vi "Example.Async.vi"() -> ()   [LabVIEW 2015, in "Inline Async Example Engine.lvlib"]
uses:
  Inline Async Example Engine.lvlib
  Inline Async APIs/VS Inline Async API/Process/Process.lvclass
  Inline Async APIs/Data Access Engine/Data Access Engine.lvclass
  Inline Async APIs/Data Access Engine/Data/Read/Read.lvclass/Read.ctl
  Inline Async APIs/Data Access Engine/Data/Write/Write.lvclass/Write.ctl
  Inline Async APIs/VS Inline Async API/Process/Process.lvclass/Process.ctl
  Inline Async APIs/Data Access Engine/Methods/Read.Data.vi
  Inline Async APIs/Data Access Engine/Methods/Write.Data.vi
  Inline Async APIs/Data Access Engine/Data/Read/Read.ProcessData.vi
  Inline Async APIs/Data Access Engine/Data/Write/Write.ProcessData.vi
  Inline Async APIs/Data Access Engine/Methods/Read.Lookup.vi
  Inline Async APIs/Data Access Engine/Methods/Write.Lookup.vi
panel:
  in  "Parameters":refnum<class "Data Access Engine.lvclass">
  in  "Process":refnum<class "Process.lvclass">
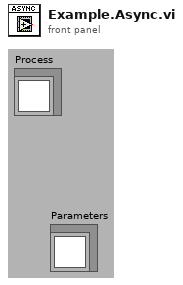
[diagram p1: front panel]
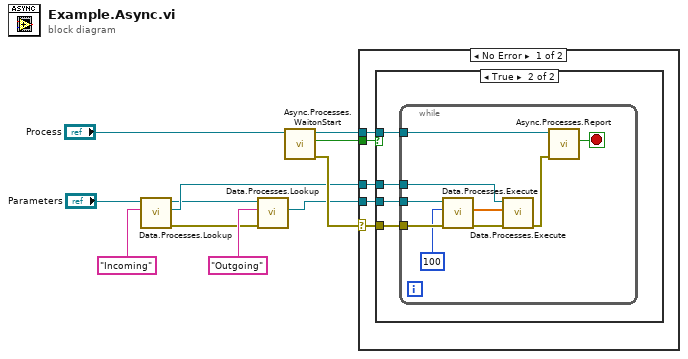
[diagram p0: block diagram]
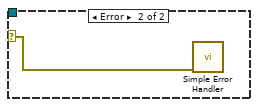
[diagram p3: hidden frame]
diagram:
  n1 = call-poly "Data.Processes.Lookup.vi"("Name"="Incoming", "Data Access API in"="Parameters") -> ("error out"=w3:errorcluster, "Ref"=w2:refnum<data-value>, "Data Access API out"=w1:refnum<class "Data Access Engine.lvclass">)  [unwired: 6 in, 1 out]
  n2 = call-poly "Data.Processes.Lookup.vi"("error in (no error)"=w3, "Name"="Outgoing", "Data Access API in"=w1) -> ("Ref"=w6:refnum<data-value>)  [unwired: 5 in, 3 out]
  n3 = call "Async.Processes.WaitonStart.vi"("Process in"="Process") -> ("error out"=w8:errorcluster, "notification"=w11:bool, "Process out"=w10:refnum<class "Process.lvclass">)  [unwired: 8 in]
  n4 = case shown="No Error" w8 {
    selector: w8 -> [w12 w30]
    tunnel: w11 -> [w16 _]
    tunnel: w10 -> [w15 _]
    tunnel: w2 -> [w14 _]
    tunnel: w6 -> [w13 _]
    frame No Error {
      n5 = case shown="True" w16 {
        tunnel: w12 -> [_ w20]
        tunnel: w15 -> [_ w19]
        tunnel: w13 -> [_ w18]
        tunnel: w14 -> [_ w17]
        frame False {
        }
        frame True {
          n6 = while {
            tunnel: w20 -> [w25]
            tunnel: w19 -> [w29]
            tunnel: w18 -> [w27]
            tunnel: w17 -> [w26]
            stop <- w28 stop-if-true
            n7 = call-poly "Data.Processes.Execute.vi"("error in (no error)"=w25, "timeout ms"=100, "Ref"=w27) -> ("error out"=w21:errorcluster, "Values"=w23:dbl[])  [unwired: 6 in, 1 out]
            n8 = call-poly "Data.Processes.Execute.vi"("error in (no error)"=w21, "Values"=w23, "Ref"=w26) -> ("error out"=w22:errorcluster)  [unwired: 8 in]
            n9 = call "Async.Processes.Report.vi"("Error"=w22, "Process in"=w29) -> ("Stop"=w28:bool)  [unwired: 8 in, 1 out]
          }
        }
      }
    }
    frame Error {
      n10 = call <vilib>:"Simple Error Handler.vi"("error in (no error)"=w30) -> ()  [unwired: 4 in, 5 out]
    }
  }
